vi "Add PUBREC.vi"(8 "error in (no error)":errorcluster, 10 "Packet Identifier":u16 format="%016b", 11 "Client ID":string) -> (0 "error out":errorcluster)   [LabVIEW 2013, in "MQTT Server.lvlib" / "StoredSessions.lvclass"]
uses:
  StoredSessions.lvclass
  Session State -- cluster.ctl
  <vilib>/LabVIEW Open Source Project/MQTT Control Packets/Control Packets/SUBSCRIBE/Topic Subscription -- cluster.ctl
  <vilib>/LabVIEW Open Source Project/MQTT Control Packets/Control Packets/ControlPacket/QualityOfService -- enum.ctl
  <vilib>/LabVIEW Open Source Project/MQTT Control Packets/Control Packets/ControlPacket/ControlPacket.lvclass
  <vilib>/LabVIEW Open Source Project/MQTT Control Packets/Control Packets/SUBSCRIBE/SUBSCRIBE.lvclass
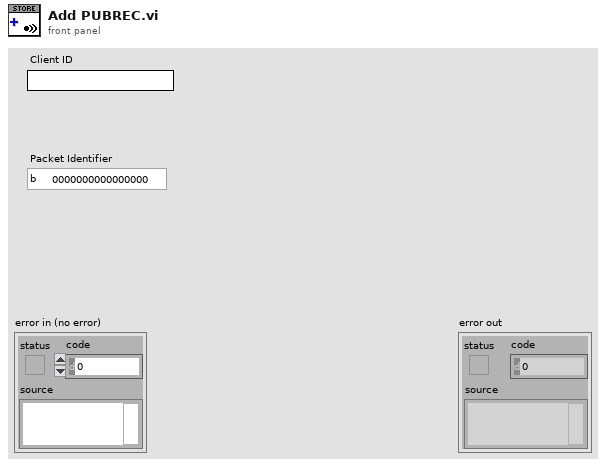
[diagram p1: front panel]
types:
  T1 = typedef "MQTT Server.lvlib/StoredSessions.lvclass/Session State -- cluster.ctl" = cluster{"Client ID":string, "Subscriptions":T2[], "PUBREC":u16[]}
  T2 = typedef "MQTT_Control_Packets.lvlib/SUBSCRIBE.lvclass/Topic Subscription -- cluster.ctl" = cluster{"Topic Filter":string, "QoS":T3}
  T3 = typedef "MQTT_Control_Packets.lvlib/ControlPacket.lvclass/QualityOfService -- enum.ctl" = enum16{"0 (At Most Once)", "1 (At Least Once)", "2 (Exactly Once)"}
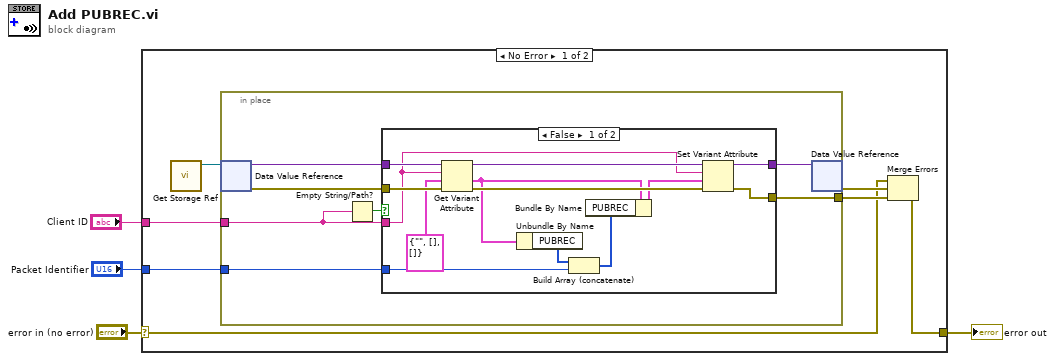
[diagram p0: block diagram]
diagram:
  n1 = case shown="No Error" "error in (no error)" {
    selector: "error in (no error)" -> [w7 w34]
    tunnel: [w6 w34] -> w3
    tunnel: "Packet Identifier" -> [w10 _]
    tunnel: "Client ID" -> [w5 _]
    frame No Error {
      n2 = call "Get Storage Ref.vi"() -> ("Storage"=w11:refnum<data-value>)  [unwired: 11 in]
      n3 = in-place {
        in-place-border: w10 -> [w12]
        in-place-border: [w16] -> w9
        in-place-border: w5 -> [w13]
        n4 = in-place-dvr #1(w11) -> (w18:variant, w15:errorcluster)
        n5 = Empty String/Path?(string/path=w13) -> (empty?=w14:bool)
        n6 = case shown="False" w14 {
          tunnel: w18 -> [w31 w33]
          tunnel: [w28 w33] -> w17
          tunnel: [w25 w32] -> w16
          tunnel: w15 -> [w30 w32]
          tunnel: w13 -> [w24 _]
          tunnel: w12 -> [w21 _]
          frame False {
            n7 = Get Variant Attribute(Variant=w31, name=w24, default value (empty Variant)=T1 {"Client ID"="", "Subscriptions"=[], "PUBREC"=[]} ("Stored Session"), error in=w30) -> (duplicate Variant=w29:variant, value=w23:T1, error out=w26:errorcluster)  [unwired: 1 out]
            n8 = Unbundle By Name(w23) -> ("PUBREC"=w22:u16[])
            n9 = Build Array (concatenate)(w22, w21) -> (w20:u16[])
            n10 = Bundle By Name(cluster=w23, "PUBREC"=w20) -> (w19:T1)
            n11 = Set Variant Attribute(Variant=w29, name=w24, value=w19, error in=w26) -> (Variant out=w28:variant, error out=w25:errorcluster)  [unwired: 1 out]
          }
          frame True {
          }
        }
        n12 = in-place-dvr #1(w17) -> (w8:errorcluster)  [unwired: 1 out]
      }
      n13 = Merge Errors(w7, w8, w9) -> (w6:errorcluster)
    }
    frame Error {
    }
  }
  "error out" <- w3
